vi "Pololu.Mgr - Disconnect.vi"(8 "error in (no error)":errorcluster, 11 "PololuCtrl in":refnum<class "PololuCtrl.lvclass">) -> (0 "error out":errorcluster, 3 "PololuCtrl out":refnum<class "PololuCtrl.lvclass">)   [LabVIEW 2018, in "PololuCtrl.lvclass"]
uses:
  PololuCtrl.lvclass
  PololuCtrl.lvclass/PololuCtrl.ctl
  Serial Port/Class/SerialPort.lvclass
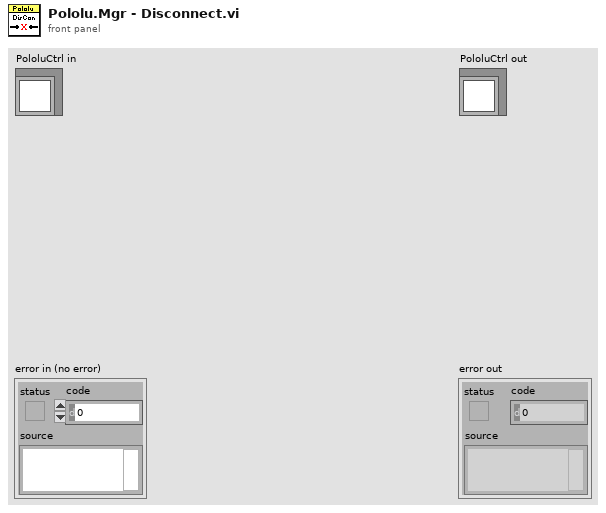
[diagram p1: front panel]
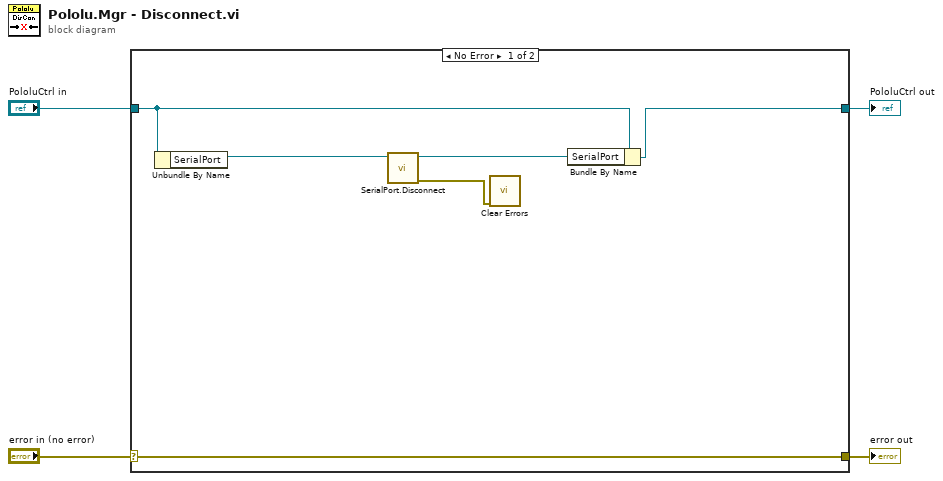
[diagram p0: block diagram]
diagram:
  n1 = case shown="No Error" "error in (no error)" {
    selector: "error in (no error)" -> [w8 w12]
    tunnel: [w8 w12] -> w3
    tunnel: [w10 w11] -> w1
    tunnel: "PololuCtrl in" -> [w9 w11]
    frame No Error {
      n2 = Unbundle By Name(w9) -> ("SerialPort"=w7:refnum<class "SerialPort.lvclass">)
      n3 = call "SerialPort.Disconnect.vi"("SerialPort in"=w7) -> ("error out"=w5:errorcluster, "SerialPort out"=w6:refnum<class "SerialPort.lvclass">)  [unwired: 8 in, 1 out]
      n4 = call <vilib>:"Clear Errors.vi"("error in (no error)"=w5) -> ()  [unwired: 5 in, 2 out]
      n5 = Bundle By Name(cluster=w9, "SerialPort"=w6) -> (w10:refnum<class "PololuCtrl.lvclass">)
    }
    frame Error {
    }
  }
  "error out" <- w3
  "PololuCtrl out" <- w1
